vi "Measurements Finished.vi"(8 "error in (no error)":errorcluster, 11 "Common Measurements in":refnum<class "Common Measurements.lvclass">) -> (0 "error out":errorcluster, 3 "Common Measurements out":refnum<class "Common Measurements.lvclass">)   [LabVIEW 2015, in "Common Measurements.lvclass"]
uses:
  Common Measurements.lvclass
  Common Measurements.lvclass/Common Measurements.ctl
  Mag Lab Measure Controller/Mag Lab Measure Controller.lvclass
  Mag Lab Error Handler/Mag Lab Error Handler.lvclass
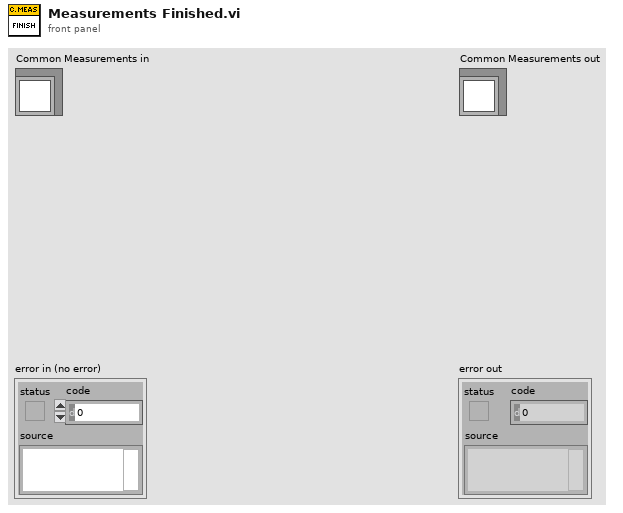
[diagram p1: front panel]
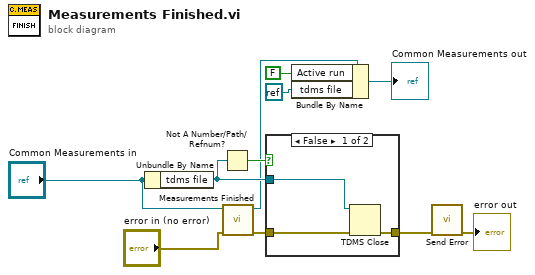
[diagram p0: block diagram]
diagram:
  n1 = Unbundle By Name("Common Measurements in") -> ("tdms file"=w9:refnum<k34>)
  n2 = Not A Number/Path/Refnum?(number/path/refnum=w9) -> (NaN/Path/Refnum?=w8:bool)
  n3 = call-parent "Measurements Finished.vi"("error in (no error)"="error in (no error)", "Mag Lab Measure Controller in"="Common Measurements in") -> ("error out"=w4:errorcluster, "Mag Lab Measure Controller out"=w1:refnum<class "Common Measurements.lvclass">)  [unwired: 8 in]
  n4 = case shown="False" w8 {
    tunnel: w9 -> [w14 _]
    tunnel: w4 -> [w13 w15]
    tunnel: [w12 w15] -> w10
    frame False {
      n5 = TDMS Close(8:w13, 11:w14) -> (0:w12:errorcluster)  [unwired: 1 out]
    }
    frame True {
    }
  }
  n6 = Bundle By Name(cluster=w1, "Active run"=FALSE, "tdms file"=refnum<k0> refnum) -> (→"Common Measurements out":refnum<class "Common Measurements.lvclass">)
  n7 = call "Send Error.vi"("error in (no error)"=w10) -> ("error out"=→"error out":errorcluster)  [unwired: 9 in, 1 out]
